vi "facade.vi"(0 "Data In":T4, 2 "Display State In":T2={"configuration visible?"=TRUE, "label visible?"=TRUE, "settings visible?"=TRUE, "start path"=path "", "path changed?"=FALSE}, 3 "Container State":T3) -> (6 "Data Out":T4, 7 "Display State Out":T2={"configuration visible?"=TRUE, "label visible?"=TRUE, "settings visible?"=TRUE, "start path"=path "", "path changed?"=FALSE}, 8 "Action":T1)   [LabVIEW 2010, in "XComponentSpecification.xctl"]
uses:
  XComponentSpecification.xctl
  data.ctl
  <vilib>/_xctls/Container State.ctl
  state.ctl
  <vilib>/_xctls/Action.ctl
  clusters/plugin_specification.ctl
  <vilib>/_xctls/XControlSupport.lvlib
panel:
  in  "label":string
  in  "settings":string(combo)
  in  "configuration":string(combo)
  in  "class":path
  # "1. Drop the controls that make up the appearance\nof the XControl here.\n\n2. Resize the window to fit the controls\n\n3. If the XControl is of fixed size,  make the \n window not resizable from VI Properties->Window Appearance.\n\n4. If you want the controls to automatically size when the XControl sizes, check  \"Scale all objects on front panel when window resizes\" in File->VI Properties->Window Size page.\n\n5. Show the block diagram and handle events for the controls on this panel."
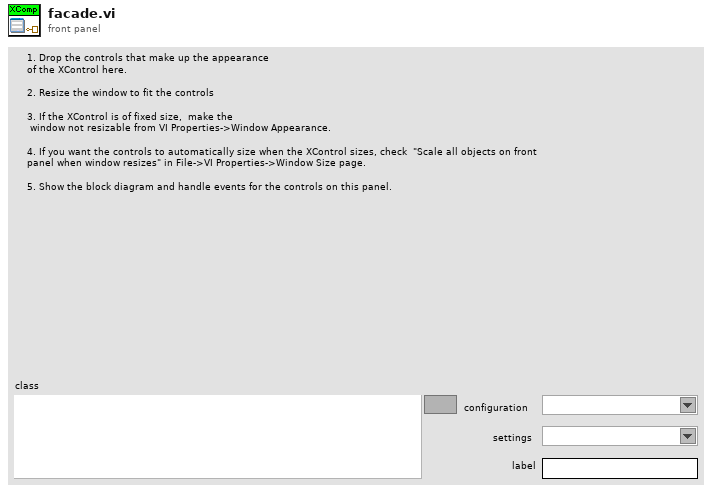
[diagram p1: front panel]
types:
  T1 = typedef "XControlSupport.lvlib/Action.ctl" = cluster{"Data Changed?":bool, "State Changed?":bool, "Action Name":string}
  T2 = typedef "XComponentSpecification.xctl/state.ctl" = cluster{"configuration visible?":bool, "label visible?":bool, "settings visible?":bool, "start path":path, "path changed?":bool}
  T3 = typedef "XControlSupport.lvlib/Container State.ctl" = cluster{"Indicator?":bool, "Run Mode?":bool, " Refnum":refnum<vi>}
  T4 = typedef "XComponentSpecification.xctl/data.ctl" = cluster{"class path":string, "configuration":string, "label":string, "settings name":string}
  T5 = enum8{"Enabled", "Disabled", "Disabled and Grayed Out"}
  T6 = typedef "plugin_specification.ctl" = cluster{"class path":string, "configuration":string, "label":string, "settings name":string}
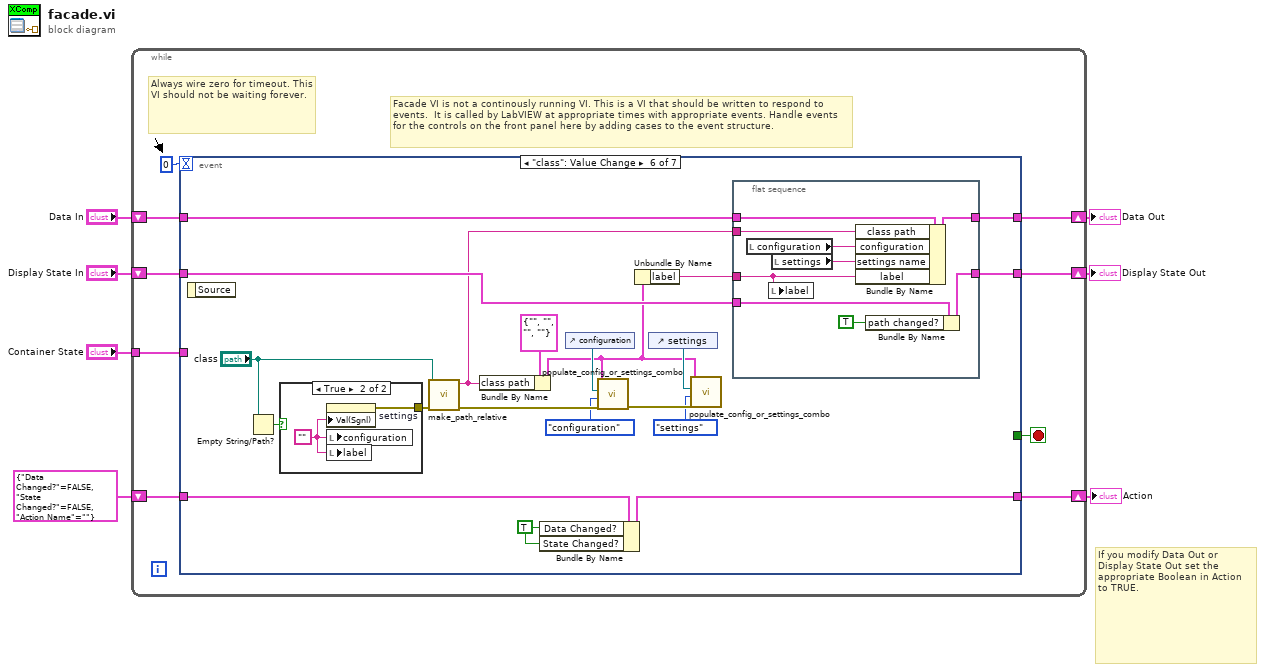
[diagram p0: block diagram]
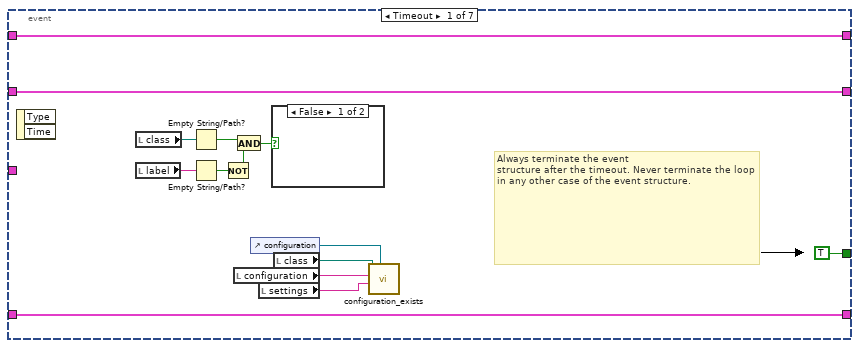
[diagram p2: hidden frame]
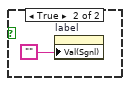
[diagram p3: hidden frame]
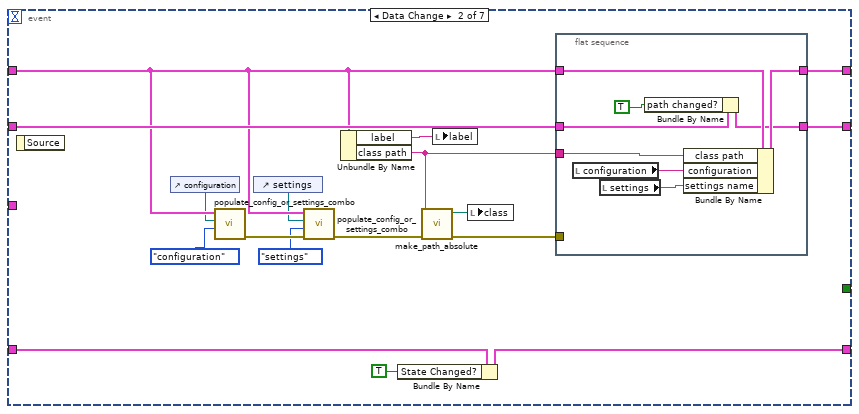
[diagram p4: hidden frame]
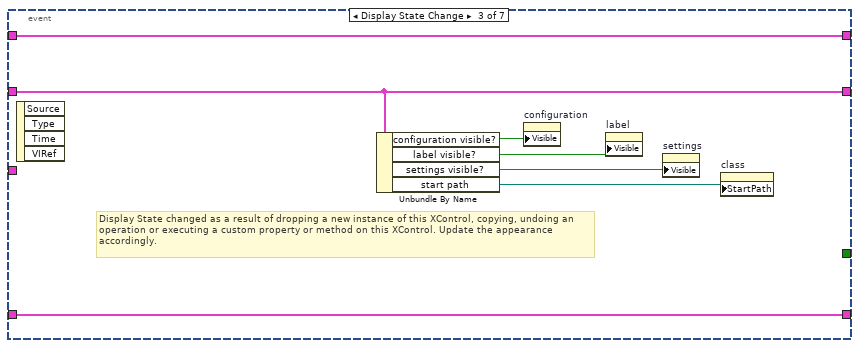
[diagram p5: hidden frame]
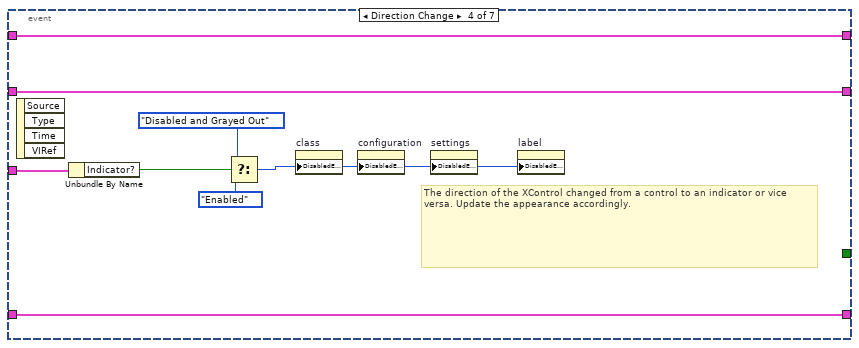
[diagram p6: hidden frame]
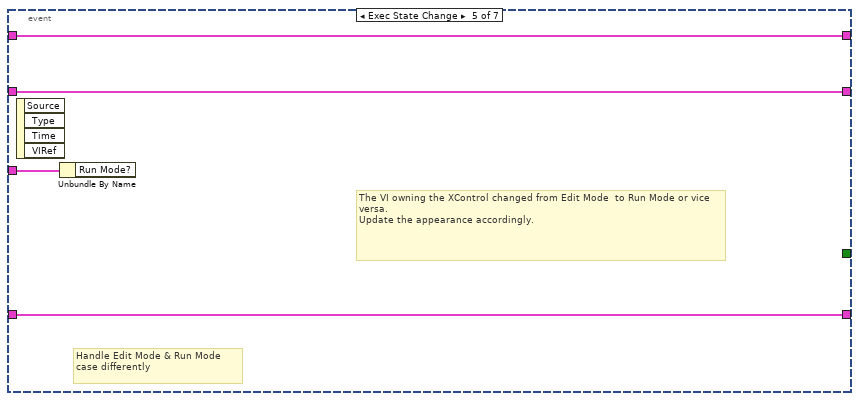
[diagram p7: hidden frame]
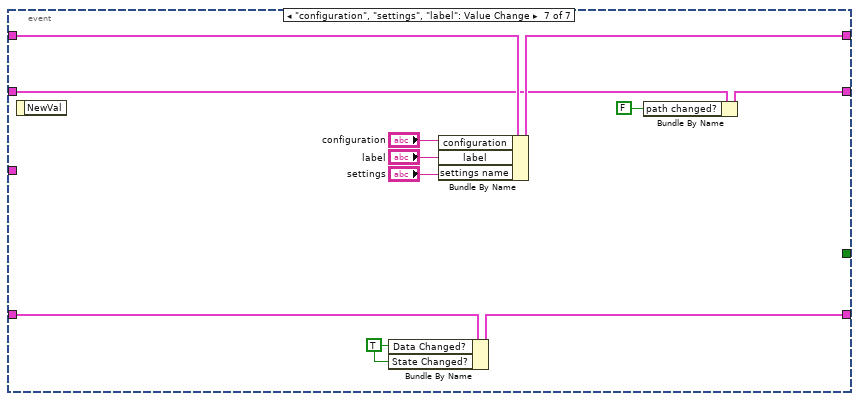
[diagram p9: hidden frame]
diagram:
  # "If you modify Data Out or\nDisplay State Out set the\nappropriate Boolean in Action\nto TRUE."
  n1 = while {
    shift-right: [w15] -> w4
    shift-left: "Display State In" -> [w16]
    tunnel: "Container State" -> [w12]
    shift-right: [w10] -> w7
    shift-left: "Data In" -> [w11]
    shift-right: [w8] -> w2
    shift-left: T1 {"Data Changed?"=FALSE, "State Changed?"=FALSE, "Action Name"=""} ("Action") -> [w9]
    stop <- w14 stop-if-true
    # "Facade VI is not a continously running VI. This is a VI that should be written to respond to events.  It is called by LabVIEW at appropriate times with appropriate events. Handle events for the controls on the front panel here by adding cases to the event structure."
    # "Always wire zero for timeout. This\nVI should not be waiting forever."
    n2 = event shown="[5] \"class\": Value Change" {
      selector: _ -> [_ _ _ _ _ _ _]
      dyn-events: _ -> [_ _ _ _ _ _ _]
      timeout: 0 -> [_ _ _ _ _ _ _]
      tunnel: w16 -> [w28 w46 w62 w70 w74 w94 w110]
      tunnel: [w28 w45 w62 w70 w74 w95 w109] -> w15
      tunnel: [TRUE _ _ _ _ _ _] -> w14
      tunnel: w12 -> [_ _ _ w71 w75 _ _]
      tunnel: w11 -> [w27 w41 w59 w69 w73 w81 w117]
      tunnel: [w27 w47 w59 w69 w73 w92 w116] -> w10
      tunnel: [w29 w33 w63 w68 w72 w89 w112] -> w8
      tunnel: w9 -> [w29 w34 w63 w68 w72 w90 w113]
      event Timeout {
        # "Always terminate the event\nstructure after the timeout. Never terminate the loop in any other case of the event structure."
        n3 = event-data() -> ()  [unwired: 1 in, 2 out]
        n4 = local read "class"() -> (w26:path)
        n5 = local read "label"() -> (w25:string)
        n6 = Empty String/Path?(string/path=w26) -> (empty?=w23:bool)
        n7 = Empty String/Path?(string/path=w25) -> (empty?=w24:bool)
        n8 = Not(x=w24) -> (.not. x?=w22:bool)
        n9 = And(x=w23, y=w22) -> (x .and. y?=w21:bool)
        n10 = local read "configuration"() -> (w18:string)
        n11 = control-ref of="configuration"() -> (w17:refnum<vi>)
        n12 = local read "settings"() -> (w19:string)
        n13 = case shown="False" w21 {
          frame False {
          }
          frame True {
            n14 = property on="label" class="Str"("Val(Sgnl)"="") -> ()  [unwired: 2 in, 2 out]
          }
        }
        n15 = local read "class"() -> (w20:path)
        n16 = call "configuration_exists.vi"(7:"configuration"=w17, "settings"=w19, 10:"configuration"=w18, "class"=w20) -> ()  [unwired: 7 in, 1 out]
      }
      event Data Change {
        n17 = event-data() -> ()  [unwired: 1 in, 1 out]
        n18 = control-ref of="configuration"() -> (w37:refnum<vi>)
        n19 = call "populate_config_or_settings_combo.vi"("type"=enum16{"configuration", "settings"}."configuration", "combo-box reference"=w37, "plug-in specification"=w41) -> ("error out"=w40:errorcluster)  [unwired: 8 in]
        n20 = control-ref of="settings"() -> (w36:refnum<vi>)
        n21 = call "populate_config_or_settings_combo.vi"("error in (no error)"=w40, "type"=enum16{"configuration", "settings"}."settings", "combo-box reference"=w36, "plug-in specification"=w41) -> ("error out"=w42:errorcluster)  [unwired: 7 in]
        n22 = Unbundle By Name(w41) -> ("label"=w32:string, "class path"=w44:string)
        n23 = Bundle By Name(cluster=w34, "State Changed?"=TRUE) -> (w33:T1)
        n24 = call "make_path_absolute.vi"("error in (no error)"=w42, "relative path"=w44) -> ("error out"=w43:errorcluster, "absolute path"=w48:path)  [unwired: 8 in]
        n25 = local write "label"(w32) -> ()
        n26 = local write "class"(w48) -> ()
        n27 = flat-sequence {
          tunnel: w46 -> [w51]
          tunnel: [w50] -> w45
          tunnel: w41 -> [w56]
          tunnel: [w54] -> w47
          tunnel: w44 -> [w53]
          tunnel: w43 -> [_]
          frame #0 {
            n28 = local read "configuration"() -> (w52:string)
            n29 = local read "settings"() -> (w55:string)
            n30 = Bundle By Name(cluster=w51, "path changed?"=TRUE) -> (w50:T2)
            n31 = Bundle By Name(cluster=w56, "class path"=w53, "configuration"=w52, "settings name"=w55) -> (w54:T4)
          }
        }
      }
      event Display State Change {
        # "Display State changed as a result of dropping a new instance of this XControl, copying, undoing an operation or executing a custom property or method on this XControl. Update the appearance accordingly."
        n32 = event-data() -> ()  [unwired: 1 in, 4 out]
        n33 = Unbundle By Name(w62) -> ("configuration visible?"=w61:bool, "label visible?"=w57:bool, "settings visible?"=w60:bool, "start path"=w58:path)
        n34 = property on="configuration" class="CmbBox"("Visible"=w61) -> ()  [unwired: 2 in, 2 out]
        n35 = property on="label" class="Str"("Visible"=w57) -> ()  [unwired: 2 in, 2 out]
        n36 = property on="settings" class="CmbBox"("Visible"=w60) -> ()  [unwired: 2 in, 2 out]
        n37 = property on="class" class="Path"("StartPath"=w58) -> ()  [unwired: 2 in, 2 out]
      }
      event Direction Change {
        # "The direction of the XControl changed from a control to an indicator or vice versa. Update the appearance accordingly."
        n38 = event-data() -> ()  [unwired: 1 in, 4 out]
        n39 = Unbundle By Name(w71) -> ("Indicator?"=w65:bool)
        n40 = Select(t=T5."Disabled and Grayed Out" ("Disabled"), s=w65, f=T5."Enabled") -> (s? t:f=w64:T5)
        n41 = property on="class" class="Path"("DisabledEnum"=w64) -> ()  [unwired: 2 in, 2 out]
        n42 = property on="configuration" class="CmbBox"("DisabledEnum"=w64) -> ()  [unwired: 2 in, 2 out]
        n43 = property on="settings" class="CmbBox"("DisabledEnum"=w64) -> ()  [unwired: 2 in, 2 out]
        n44 = property on="label" class="Str"("DisabledEnum"=w64) -> ()  [unwired: 2 in, 2 out]
      }
      event Exec State Change {
        # "The VI owning the XControl changed from Edit Mode  to Run Mode or vice versa.\nUpdate the appearance accordingly."
        # "Handle Edit Mode & Run Mode\ncase differently"
        n45 = event-data() -> ()  [unwired: 1 in, 4 out]
        n46 = Unbundle By Name(w75) -> ()  [unwired: 1 out]
      }
      event "class": Value Change {
        w82 = TRUE ("Data Changed?")
        n47 = event-data() -> ()  [unwired: 1 in, 1 out]
        n48 = Empty String/Path?(string/path="class") -> (empty?=w76:bool)
        n49 = case shown="True" w76 {
          tunnel: [_ w97] -> w77
          frame False {
          }
          frame True {
            w96 = ""
            n50 = property on="settings" class="CmbBox"("Val(Sgnl)"=w96) -> (error out=w97:errorcluster)  [unwired: 2 in, 1 out]
            n51 = local write "configuration"(w96) -> ()
            n52 = local write "label"(w96) -> ()
          }
        }
        n53 = call "make_path_relative.vi"("error in (no error)"=w77, "absolute path"="class") -> ("error out"=w88:errorcluster, "relative path"=w91:string)  [unwired: 8 in]
        n54 = Bundle By Name(cluster=T6 {"class path"="", "configuration"="", "label"="", "settings name"=""} ("plug-in specification"), "class path"=w91) -> (w80:T6)
        n55 = Bundle By Name(cluster=w90, "Data Changed?"=w82, "State Changed?"=w82) -> (w89:T1)
        n56 = control-ref of="configuration"() -> (w87:refnum<vi>)
        n57 = call "populate_config_or_settings_combo.vi"("error in (no error)"=w88, "type"=enum16{"configuration", "settings"}."configuration", "combo-box reference"=w87, "plug-in specification"=w80) -> ("error out"=w85:errorcluster)  [unwired: 7 in]
        n58 = Unbundle By Name(w80) -> ("label"=w79:string)
        n59 = control-ref of="settings"() -> (w83:refnum<vi>)
        n60 = call "populate_config_or_settings_combo.vi"("error in (no error)"=w85, "type"=enum16{"configuration", "settings"}."settings", "combo-box reference"=w83, "plug-in specification"=w80) -> ()  [unwired: 7 in, 1 out]
        n61 = flat-sequence {
          tunnel: w94 -> [w100]
          tunnel: [w99] -> w95
          tunnel: w81 -> [w106]
          tunnel: [w105] -> w92
          tunnel: w91 -> [w104]
          tunnel: w79 -> [w98]
          frame #0 {
            n62 = local read "configuration"() -> (w103:string)
            n63 = local write "label"(w98) -> ()
            n64 = local read "settings"() -> (w102:string)
            n65 = Bundle By Name(cluster=w106, "class path"=w104, "configuration"=w103, "settings name"=w102, "label"=w98) -> (w105:T4)
            n66 = Bundle By Name(cluster=w100, "path changed?"=TRUE) -> (w99:T2)
          }
        }
      }
      event "configuration", "settings", "label": Value Change {
        w107 = TRUE ("Data Changed?")
        n67 = event-data() -> ()  [unwired: 1 in, 1 out]
        n68 = Bundle By Name(cluster=w113, "Data Changed?"=w107, "State Changed?"=w107) -> (w112:T1)
        n69 = Bundle By Name(cluster=w117, "configuration"="configuration", "label"="label", "settings name"="settings") -> (w116:T4)
        n70 = Bundle By Name(cluster=w110, "path changed?"=FALSE) -> (w109:T2)
      }
    }
  }
  "Display State Out" <- w4
  "Data Out" <- w7
  "Action" <- w2
